vi "Sample_application.vi"() -> ()   [LabVIEW 2026]
uses:
  x64/Release/CanSharkApi_Dll1.dll
panel:
  in  "datalog":bool
  out "?":string="CAN Shark API's for Classic CAN & CANFD communication"
  in  "error in":errorcluster
  out "Serial Number":u32[](array[numeric])
  out "Device Path":string[](array[string])
  out "Connected Devices":string
  out "?":string="CAN Shark API's for Classic CAN & CANFD communication"
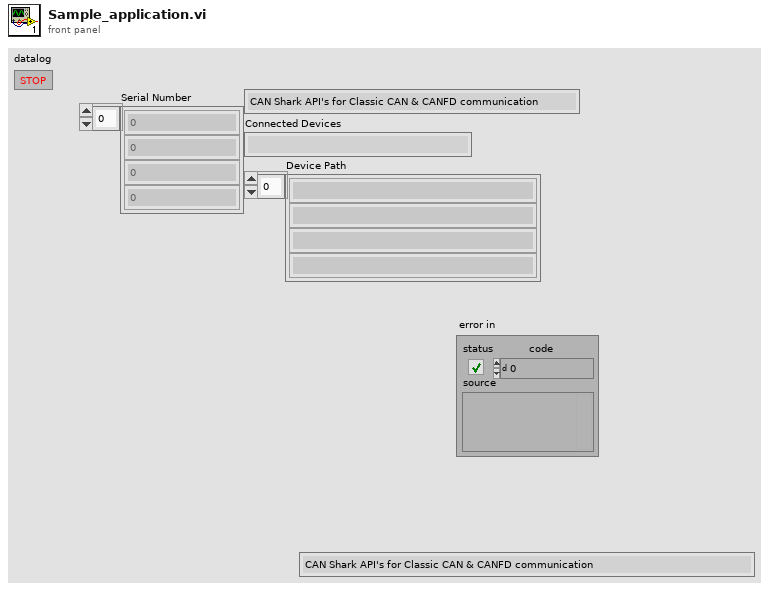
[diagram p1: front panel]
types:
  T1 = cluster{"cluster":cluster{"initialized array[0]":u16, "initialized array[1]":u16, "initialized array[2]":u16, "initialized array[3]":u16, "initialized array[4]":u16, "initialized array[5]":u16, "initialized array[6]":u16, "initialized array[7]":u16, "initialized array[8]":u16, "initialized array[9]":u16, "initialized array[10]":u16, "initialized array[11]":u16, "initialized array[12]":u16, "initialized array[13]":u16, "initialized array[14]":u16, "initialized array[15]":u16, "initialized array[16]":u16, "initialized array[17]":u16, "initialized array[18]":u16, "initialized array[19]":u16, "initialized array[20]":u16, "initialized array[21]":u16, "initialized array[22]":u16, "initialized array[23]":u16, "initialized array[24]":u16, "initialized array[25]":u16, "initialized array[26]":u16, "initialized array[27]":u16, "initialized array[28]":u16, "initialized array[29]":u16, "initialized array[30]":u16, "initialized array[31]":u16, "initialized array[32]":u16, "initialized array[33]":u16, "initialized array[34]":u16, "initialized array[35]":u16, "initialized array[36]":u16, "initialized array[37]":u16, "initialized array[38]":u16, "initialized array[39]":u16, "initialized array[40]":u16, "initialized array[41]":u16, "initialized array[42]":u16, "initialized array[43]":u16, "initialized array[44]":u16, "initialized array[45]":u16, "initialized array[46]":u16, "initialized array[47]":u16, "initialized array[48]":u16, "initialized array[49]":u16, "initialized array[50]":u16, "initialized array[51]":u16, "initialized array[52]":u16, "initialized array[53]":u16, "initialized array[54]":u16, "initialized array[55]":u16, "initialized array[56]":u16, "initialized array[57]":u16, "initialized array[58]":u16, "initialized array[59]":u16, "initialized array[60]":u16, "initialized array[61]":u16, "initialized array[62]":u16, "initialized array[63]":u16, "initialized array[64]":u16, "initialized array[65]":u16, "initialized array[66]":u16, "initialized array[67]":u16, "initialized array[68]":u16, "initialized array[69]":u16, "initialized array[70]":u16, "initialized array[71]":u16, "initialized array[72]":u16, "initialized array[73]":u16, "initialized array[74]":u16, "initialized array[75]":u16, "initialized array[76]":u16, "initialized array[77]":u16, "initialized array[78]":u16, "initialized array[79]":u16, "initialized array[80]":u16, "initialized array[81]":u16, "initialized array[82]":u16, "initialized array[83]":u16, "initialized array[84]":u16, "initialized array[85]":u16, "initialized array[86]":u16, "initialized array[87]":u16, "initialized array[88]":u16, "initialized array[89]":u16, "initialized array[90]":u16, "initialized array[91]":u16, "initialized array[92]":u16, "initialized array[93]":u16, "initialized array[94]":u16, "initialized array[95]":u16, "initialized array[96]":u16, "initialized array[97]":u16, "initialized array[98]":u16, "initialized array[99]":u16, "initialized array[100]":u16, "initialized array[101]":u16, "initialized array[102]":u16, "initialized array[103]":u16, "initialized array[104]":u16, "initialized array[105]":u16, "initialized array[106]":u16, "initialized array[107]":u16, "initialized array[108]":u16, "initialized array[109]":u16, "initialized array[110]":u16, "initialized array[111]":u16, "initialized array[112]":u16, "initialized array[113]":u16, "initialized array[114]":u16, "initialized array[115]":u16, "initialized array[116]":u16, "initialized array[117]":u16, "initialized array[118]":u16, "initialized array[119]":u16, "initialized array[120]":u16, "initialized array[121]":u16, "initialized array[122]":u16, "initialized array[123]":u16, "initialized array[124]":u16, "initialized array[125]":u16, "initialized array[126]":u16, "initialized array[127]":u16, "initialized array[128]":u16, "initialized array[129]":u16, "initialized array[130]":u16, "initialized array[131]":u16, "initialized array[132]":u16, "initialized array[133]":u16, "initialized array[134]":u16, "initialized array[135]":u16, "initialized array[136]":u16, "initialized array[137]":u16, "initialized array[138]":u16, "initialized array[139]":u16, "initialized array[140]":u16, "initialized array[141]":u16, "initialized array[142]":u16, "initialized array[143]":u16, "initialized array[144]":u16, "initialized array[145]":u16, "initialized array[146]":u16, "initialized array[147]":u16, "initialized array[148]":u16, "initialized array[149]":u16, "initialized array[150]":u16, "initialized array[151]":u16, "initialized array[152]":u16, "initialized array[153]":u16, "initialized array[154]":u16, "initialized array[155]":u16, "initialized array[156]":u16, "initialized array[157]":u16, "initialized array[158]":u16, "initialized array[159]":u16, "initialized array[160]":u16, "initialized array[161]":u16, "initialized array[162]":u16, "initialized array[163]":u16, "initialized array[164]":u16, "initialized array[165]":u16, "initialized array[166]":u16, "initialized array[167]":u16, "initialized array[168]":u16, "initialized array[169]":u16, "initialized array[170]":u16, "initialized array[171]":u16, "initialized array[172]":u16, "initialized array[173]":u16, "initialized array[174]":u16, "initialized array[175]":u16, "initialized array[176]":u16, "initialized array[177]":u16, "initialized array[178]":u16, "initialized array[179]":u16, "initialized array[180]":u16, "initialized array[181]":u16, "initialized array[182]":u16, "initialized array[183]":u16, "initialized array[184]":u16, "initialized array[185]":u16, "initialized array[186]":u16, "initialized array[187]":u16, "initialized array[188]":u16, "initialized array[189]":u16, "initialized array[190]":u16, "initialized array[191]":u16, "initialized array[192]":u16, "initialized array[193]":u16, "initialized array[194]":u16, "initialized array[195]":u16, "initialized array[196]":u16, "initialized array[197]":u16, "initialized array[198]":u16, "initialized array[199]":u16, "initialized array[200]":u16, "initialized array[201]":u16, "initialized array[202]":u16, "initialized array[203]":u16, "initialized array[204]":u16, "initialized array[205]":u16, "initialized array[206]":u16, "initialized array[207]":u16, "initialized array[208]":u16, "initialized array[209]":u16, "initialized array[210]":u16, "initialized array[211]":u16, "initialized array[212]":u16, "initialized array[213]":u16, "initialized array[214]":u16, "initialized array[215]":u16, "initialized array[216]":u16, "initialized array[217]":u16, "initialized array[218]":u16, "initialized array[219]":u16, "initialized array[220]":u16, "initialized array[221]":u16, "initialized array[222]":u16, "initialized array[223]":u16, "initialized array[224]":u16, "initialized array[225]":u16, "initialized array[226]":u16, "initialized array[227]":u16, "initialized array[228]":u16, "initialized array[229]":u16, "initialized array[230]":u16, "initialized array[231]":u16, "initialized array[232]":u16, "initialized array[233]":u16, "initialized array[234]":u16, "initialized array[235]":u16, "initialized array[236]":u16, "initialized array[237]":u16, "initialized array[238]":u16, "initialized array[239]":u16, "initialized array[240]":u16, "initialized array[241]":u16, "initialized array[242]":u16, "initialized array[243]":u16, "initialized array[244]":u16, "initialized array[245]":u16, "initialized array[246]":u16, "initialized array[247]":u16, "initialized array[248]":u16, "initialized array[249]":u16, "initialized array[250]":u16, "initialized array[251]":u16, "initialized array[252]":u16, "initialized array[253]":u16, "initialized array[254]":u16, "initialized array[255]":u16}, "Serial Number":u32}[]
  T2 = cluster{"cluster":cluster{"initialized array[0]":u16, "initialized array[1]":u16, "initialized array[2]":u16, "initialized array[3]":u16, "initialized array[4]":u16, "initialized array[5]":u16, "initialized array[6]":u16, "initialized array[7]":u16, "initialized array[8]":u16, "initialized array[9]":u16, "initialized array[10]":u16, "initialized array[11]":u16, "initialized array[12]":u16, "initialized array[13]":u16, "initialized array[14]":u16, "initialized array[15]":u16, "initialized array[16]":u16, "initialized array[17]":u16, "initialized array[18]":u16, "initialized array[19]":u16, "initialized array[20]":u16, "initialized array[21]":u16, "initialized array[22]":u16, "initialized array[23]":u16, "initialized array[24]":u16, "initialized array[25]":u16, "initialized array[26]":u16, "initialized array[27]":u16, "initialized array[28]":u16, "initialized array[29]":u16, "initialized array[30]":u16, "initialized array[31]":u16, "initialized array[32]":u16, "initialized array[33]":u16, "initialized array[34]":u16, "initialized array[35]":u16, "initialized array[36]":u16, "initialized array[37]":u16, "initialized array[38]":u16, "initialized array[39]":u16, "initialized array[40]":u16, "initialized array[41]":u16, "initialized array[42]":u16, "initialized array[43]":u16, "initialized array[44]":u16, "initialized array[45]":u16, "initialized array[46]":u16, "initialized array[47]":u16, "initialized array[48]":u16, "initialized array[49]":u16, "initialized array[50]":u16, "initialized array[51]":u16, "initialized array[52]":u16, "initialized array[53]":u16, "initialized array[54]":u16, "initialized array[55]":u16, "initialized array[56]":u16, "initialized array[57]":u16, "initialized array[58]":u16, "initialized array[59]":u16, "initialized array[60]":u16, "initialized array[61]":u16, "initialized array[62]":u16, "initialized array[63]":u16, "initialized array[64]":u16, "initialized array[65]":u16, "initialized array[66]":u16, "initialized array[67]":u16, "initialized array[68]":u16, "initialized array[69]":u16, "initialized array[70]":u16, "initialized array[71]":u16, "initialized array[72]":u16, "initialized array[73]":u16, "initialized array[74]":u16, "initialized array[75]":u16, "initialized array[76]":u16, "initialized array[77]":u16, "initialized array[78]":u16, "initialized array[79]":u16, "initialized array[80]":u16, "initialized array[81]":u16, "initialized array[82]":u16, "initialized array[83]":u16, "initialized array[84]":u16, "initialized array[85]":u16, "initialized array[86]":u16, "initialized array[87]":u16, "initialized array[88]":u16, "initialized array[89]":u16, "initialized array[90]":u16, "initialized array[91]":u16, "initialized array[92]":u16, "initialized array[93]":u16, "initialized array[94]":u16, "initialized array[95]":u16, "initialized array[96]":u16, "initialized array[97]":u16, "initialized array[98]":u16, "initialized array[99]":u16, "initialized array[100]":u16, "initialized array[101]":u16, "initialized array[102]":u16, "initialized array[103]":u16, "initialized array[104]":u16, "initialized array[105]":u16, "initialized array[106]":u16, "initialized array[107]":u16, "initialized array[108]":u16, "initialized array[109]":u16, "initialized array[110]":u16, "initialized array[111]":u16, "initialized array[112]":u16, "initialized array[113]":u16, "initialized array[114]":u16, "initialized array[115]":u16, "initialized array[116]":u16, "initialized array[117]":u16, "initialized array[118]":u16, "initialized array[119]":u16, "initialized array[120]":u16, "initialized array[121]":u16, "initialized array[122]":u16, "initialized array[123]":u16, "initialized array[124]":u16, "initialized array[125]":u16, "initialized array[126]":u16, "initialized array[127]":u16, "initialized array[128]":u16, "initialized array[129]":u16, "initialized array[130]":u16, "initialized array[131]":u16, "initialized array[132]":u16, "initialized array[133]":u16, "initialized array[134]":u16, "initialized array[135]":u16, "initialized array[136]":u16, "initialized array[137]":u16, "initialized array[138]":u16, "initialized array[139]":u16, "initialized array[140]":u16, "initialized array[141]":u16, "initialized array[142]":u16, "initialized array[143]":u16, "initialized array[144]":u16, "initialized array[145]":u16, "initialized array[146]":u16, "initialized array[147]":u16, "initialized array[148]":u16, "initialized array[149]":u16, "initialized array[150]":u16, "initialized array[151]":u16, "initialized array[152]":u16, "initialized array[153]":u16, "initialized array[154]":u16, "initialized array[155]":u16, "initialized array[156]":u16, "initialized array[157]":u16, "initialized array[158]":u16, "initialized array[159]":u16, "initialized array[160]":u16, "initialized array[161]":u16, "initialized array[162]":u16, "initialized array[163]":u16, "initialized array[164]":u16, "initialized array[165]":u16, "initialized array[166]":u16, "initialized array[167]":u16, "initialized array[168]":u16, "initialized array[169]":u16, "initialized array[170]":u16, "initialized array[171]":u16, "initialized array[172]":u16, "initialized array[173]":u16, "initialized array[174]":u16, "initialized array[175]":u16, "initialized array[176]":u16, "initialized array[177]":u16, "initialized array[178]":u16, "initialized array[179]":u16, "initialized array[180]":u16, "initialized array[181]":u16, "initialized array[182]":u16, "initialized array[183]":u16, "initialized array[184]":u16, "initialized array[185]":u16, "initialized array[186]":u16, "initialized array[187]":u16, "initialized array[188]":u16, "initialized array[189]":u16, "initialized array[190]":u16, "initialized array[191]":u16, "initialized array[192]":u16, "initialized array[193]":u16, "initialized array[194]":u16, "initialized array[195]":u16, "initialized array[196]":u16, "initialized array[197]":u16, "initialized array[198]":u16, "initialized array[199]":u16, "initialized array[200]":u16, "initialized array[201]":u16, "initialized array[202]":u16, "initialized array[203]":u16, "initialized array[204]":u16, "initialized array[205]":u16, "initialized array[206]":u16, "initialized array[207]":u16, "initialized array[208]":u16, "initialized array[209]":u16, "initialized array[210]":u16, "initialized array[211]":u16, "initialized array[212]":u16, "initialized array[213]":u16, "initialized array[214]":u16, "initialized array[215]":u16, "initialized array[216]":u16, "initialized array[217]":u16, "initialized array[218]":u16, "initialized array[219]":u16, "initialized array[220]":u16, "initialized array[221]":u16, "initialized array[222]":u16, "initialized array[223]":u16, "initialized array[224]":u16, "initialized array[225]":u16, "initialized array[226]":u16, "initialized array[227]":u16, "initialized array[228]":u16, "initialized array[229]":u16, "initialized array[230]":u16, "initialized array[231]":u16, "initialized array[232]":u16, "initialized array[233]":u16, "initialized array[234]":u16, "initialized array[235]":u16, "initialized array[236]":u16, "initialized array[237]":u16, "initialized array[238]":u16, "initialized array[239]":u16, "initialized array[240]":u16, "initialized array[241]":u16, "initialized array[242]":u16, "initialized array[243]":u16, "initialized array[244]":u16, "initialized array[245]":u16, "initialized array[246]":u16, "initialized array[247]":u16, "initialized array[248]":u16, "initialized array[249]":u16, "initialized array[250]":u16, "initialized array[251]":u16, "initialized array[252]":u16, "initialized array[253]":u16, "initialized array[254]":u16, "initialized array[255]":u16}, "Serial Number":u32}
  T3 = cluster{"initialized array[0]":u16, "initialized array[1]":u16, "initialized array[2]":u16, "initialized array[3]":u16, "initialized array[4]":u16, "initialized array[5]":u16, "initialized array[6]":u16, "initialized array[7]":u16, "initialized array[8]":u16, "initialized array[9]":u16, "initialized array[10]":u16, "initialized array[11]":u16, "initialized array[12]":u16, "initialized array[13]":u16, "initialized array[14]":u16, "initialized array[15]":u16, "initialized array[16]":u16, "initialized array[17]":u16, "initialized array[18]":u16, "initialized array[19]":u16, "initialized array[20]":u16, "initialized array[21]":u16, "initialized array[22]":u16, "initialized array[23]":u16, "initialized array[24]":u16, "initialized array[25]":u16, "initialized array[26]":u16, "initialized array[27]":u16, "initialized array[28]":u16, "initialized array[29]":u16, "initialized array[30]":u16, "initialized array[31]":u16, "initialized array[32]":u16, "initialized array[33]":u16, "initialized array[34]":u16, "initialized array[35]":u16, "initialized array[36]":u16, "initialized array[37]":u16, "initialized array[38]":u16, "initialized array[39]":u16, "initialized array[40]":u16, "initialized array[41]":u16, "initialized array[42]":u16, "initialized array[43]":u16, "initialized array[44]":u16, "initialized array[45]":u16, "initialized array[46]":u16, "initialized array[47]":u16, "initialized array[48]":u16, "initialized array[49]":u16, "initialized array[50]":u16, "initialized array[51]":u16, "initialized array[52]":u16, "initialized array[53]":u16, "initialized array[54]":u16, "initialized array[55]":u16, "initialized array[56]":u16, "initialized array[57]":u16, "initialized array[58]":u16, "initialized array[59]":u16, "initialized array[60]":u16, "initialized array[61]":u16, "initialized array[62]":u16, "initialized array[63]":u16, "initialized array[64]":u16, "initialized array[65]":u16, "initialized array[66]":u16, "initialized array[67]":u16, "initialized array[68]":u16, "initialized array[69]":u16, "initialized array[70]":u16, "initialized array[71]":u16, "initialized array[72]":u16, "initialized array[73]":u16, "initialized array[74]":u16, "initialized array[75]":u16, "initialized array[76]":u16, "initialized array[77]":u16, "initialized array[78]":u16, "initialized array[79]":u16, "initialized array[80]":u16, "initialized array[81]":u16, "initialized array[82]":u16, "initialized array[83]":u16, "initialized array[84]":u16, "initialized array[85]":u16, "initialized array[86]":u16, "initialized array[87]":u16, "initialized array[88]":u16, "initialized array[89]":u16, "initialized array[90]":u16, "initialized array[91]":u16, "initialized array[92]":u16, "initialized array[93]":u16, "initialized array[94]":u16, "initialized array[95]":u16, "initialized array[96]":u16, "initialized array[97]":u16, "initialized array[98]":u16, "initialized array[99]":u16, "initialized array[100]":u16, "initialized array[101]":u16, "initialized array[102]":u16, "initialized array[103]":u16, "initialized array[104]":u16, "initialized array[105]":u16, "initialized array[106]":u16, "initialized array[107]":u16, "initialized array[108]":u16, "initialized array[109]":u16, "initialized array[110]":u16, "initialized array[111]":u16, "initialized array[112]":u16, "initialized array[113]":u16, "initialized array[114]":u16, "initialized array[115]":u16, "initialized array[116]":u16, "initialized array[117]":u16, "initialized array[118]":u16, "initialized array[119]":u16, "initialized array[120]":u16, "initialized array[121]":u16, "initialized array[122]":u16, "initialized array[123]":u16, "initialized array[124]":u16, "initialized array[125]":u16, "initialized array[126]":u16, "initialized array[127]":u16, "initialized array[128]":u16, "initialized array[129]":u16, "initialized array[130]":u16, "initialized array[131]":u16, "initialized array[132]":u16, "initialized array[133]":u16, "initialized array[134]":u16, "initialized array[135]":u16, "initialized array[136]":u16, "initialized array[137]":u16, "initialized array[138]":u16, "initialized array[139]":u16, "initialized array[140]":u16, "initialized array[141]":u16, "initialized array[142]":u16, "initialized array[143]":u16, "initialized array[144]":u16, "initialized array[145]":u16, "initialized array[146]":u16, "initialized array[147]":u16, "initialized array[148]":u16, "initialized array[149]":u16, "initialized array[150]":u16, "initialized array[151]":u16, "initialized array[152]":u16, "initialized array[153]":u16, "initialized array[154]":u16, "initialized array[155]":u16, "initialized array[156]":u16, "initialized array[157]":u16, "initialized array[158]":u16, "initialized array[159]":u16, "initialized array[160]":u16, "initialized array[161]":u16, "initialized array[162]":u16, "initialized array[163]":u16, "initialized array[164]":u16, "initialized array[165]":u16, "initialized array[166]":u16, "initialized array[167]":u16, "initialized array[168]":u16, "initialized array[169]":u16, "initialized array[170]":u16, "initialized array[171]":u16, "initialized array[172]":u16, "initialized array[173]":u16, "initialized array[174]":u16, "initialized array[175]":u16, "initialized array[176]":u16, "initialized array[177]":u16, "initialized array[178]":u16, "initialized array[179]":u16, "initialized array[180]":u16, "initialized array[181]":u16, "initialized array[182]":u16, "initialized array[183]":u16, "initialized array[184]":u16, "initialized array[185]":u16, "initialized array[186]":u16, "initialized array[187]":u16, "initialized array[188]":u16, "initialized array[189]":u16, "initialized array[190]":u16, "initialized array[191]":u16, "initialized array[192]":u16, "initialized array[193]":u16, "initialized array[194]":u16, "initialized array[195]":u16, "initialized array[196]":u16, "initialized array[197]":u16, "initialized array[198]":u16, "initialized array[199]":u16, "initialized array[200]":u16, "initialized array[201]":u16, "initialized array[202]":u16, "initialized array[203]":u16, "initialized array[204]":u16, "initialized array[205]":u16, "initialized array[206]":u16, "initialized array[207]":u16, "initialized array[208]":u16, "initialized array[209]":u16, "initialized array[210]":u16, "initialized array[211]":u16, "initialized array[212]":u16, "initialized array[213]":u16, "initialized array[214]":u16, "initialized array[215]":u16, "initialized array[216]":u16, "initialized array[217]":u16, "initialized array[218]":u16, "initialized array[219]":u16, "initialized array[220]":u16, "initialized array[221]":u16, "initialized array[222]":u16, "initialized array[223]":u16, "initialized array[224]":u16, "initialized array[225]":u16, "initialized array[226]":u16, "initialized array[227]":u16, "initialized array[228]":u16, "initialized array[229]":u16, "initialized array[230]":u16, "initialized array[231]":u16, "initialized array[232]":u16, "initialized array[233]":u16, "initialized array[234]":u16, "initialized array[235]":u16, "initialized array[236]":u16, "initialized array[237]":u16, "initialized array[238]":u16, "initialized array[239]":u16, "initialized array[240]":u16, "initialized array[241]":u16, "initialized array[242]":u16, "initialized array[243]":u16, "initialized array[244]":u16, "initialized array[245]":u16, "initialized array[246]":u16, "initialized array[247]":u16, "initialized array[248]":u16, "initialized array[249]":u16, "initialized array[250]":u16, "initialized array[251]":u16, "initialized array[252]":u16, "initialized array[253]":u16, "initialized array[254]":u16, "initialized array[255]":u16}
  T4 = cluster{"DeviceIndex":i32, "Mode":i32, "BaudRate":i32, "DataBitRate":i32}[]
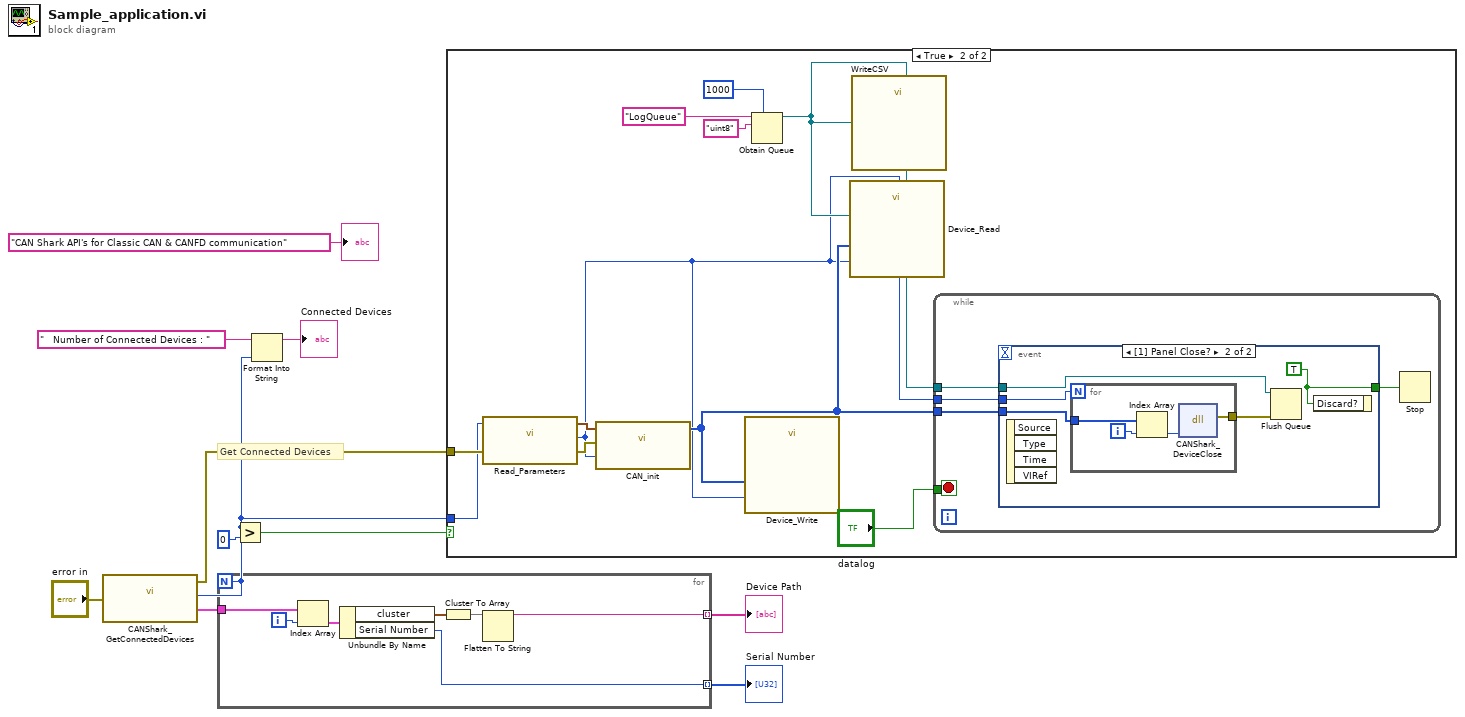
[diagram p0: block diagram]
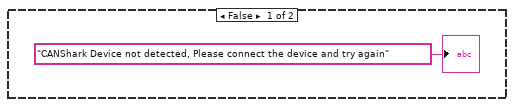
[diagram p2: hidden frame]
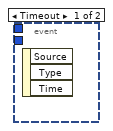
[diagram p3: hidden frame]
diagram:
  # "Get Connected Devices"
  n1 = call "CANShark_GetConnectedDevices.vi"("error in (no error)"="error in") -> ("deviceList"=w5:T1, "Connected Devices"=w1:u8, "error out"=w3:errorcluster)  [unwired: 8 in]
  n2 = for {
    N: w1 -> [_]
    tunnel: [w15] -> w7 mode=indexing
    tunnel: [w14] -> w8 mode=indexing
    tunnel: w5 -> [w12]
    i -> [w18]
    n3 = Index Array(array=w12, index=w18) -> (element=w13:T2)
    n4 = Unbundle By Name(w13) -> ("cluster"=w17:T3, "Serial Number"=w15:u32)
    n5 = Cluster To Array(cluster=w17) -> (array=w16:u16[])
    n6 = Flatten To String(anything=w16) -> (data string=w14:string)  [unwired: 3 in, 2 out]
  }
  "Device Path" <- w8
  "Serial Number" <- w7
  n7 = Greater?(x=w1, y=u8 0) -> (0:w2:bool)
  n8 = Format Into String(initial string="   Number of Connected Devices : ", w1) -> (resulting string=→"Connected Devices":string)  [unwired: 2 in, 1 out]
  n9 = case shown="True" w2 {
    tunnel: w3 -> [_ w28]
    tunnel: w1 -> [_ w27]
    frame False {
      "?" <- "CANShark Device not detected, Please connect the device and try again"
    }
    frame True {
      n10 = call "Read_Parameters.vi"("error in"=w28, "device count"=w27) -> ("error out"=w29:errorcluster, "Selected Devices"=w20:i32, "Device Configuration"=w30:T4)  [unwired: 7 in]
      n11 = call "CAN_init.vi"("Selected Count"=w20, "error in (no error)"=w29, "DEVICE CONFIG"=w30) -> ("Device Handler"=w25:i64[])  [unwired: 7 in, 1 out]
      n12 = call "Device_Write.vi"("Device Handler pointers"=w25, "Selected Device count"=w20) -> ()  [unwired: 10 in]
      n13 = Obtain Queue(max queue size (-1, unlimited)=1000, name (unnamed)="LogQueue", element data type="uint8") -> (queue out=w21:refnum<queue>)  [unwired: 2 in, 2 out]
      n14 = call "Device_Read.vi"("queue out"=w21, "Selected Count"=w20, "Device Handler pointer"=w25) -> ()  [unwired: 9 in]
      n15 = call "WriteCSV.vi"("Log Queue"=w21) -> ()  [unwired: 9 in, 2 out]
      n16 = while {
        tunnel: w25 -> [w35]
        tunnel: w20 -> [w34]
        tunnel: "datalog" -> [w33]
        tunnel: w21 -> [w31]
        stop <- w33 stop-if-true
        n17 = event shown="[1] Panel Close?" {
          selector: _ -> [_ _]
          dyn-events: _ -> [_ _]
          timeout: _ -> [_ _]
          tunnel: w35 -> [_ w39]
          tunnel: w34 -> [_ w40]
          tunnel: [_ w38] -> w32
          tunnel: w31 -> [_ w36]
          event Timeout {
            n18 = event-data() -> ()  [unwired: 1 in, 3 out]
          }
          event Panel Close? {
            w38 = TRUE
            n19 = event-data() -> ()  [unwired: 1 in, 4 out]
            n20 = for {
              N: w40 -> [_]
              tunnel: w39 -> [w42]
              tunnel: [w41] -> w37
              i -> [w43]
              n21 = Index Array(array=w42, index=w43) -> (element=w44:i64)
              n22 = dll-call lib="C:/Users/TECQNIO/Documents/CANSHARK LABVIEW API PACKAGE/x64/Release/CanSharkApi_Dll1.dll" fn="CANShark_DeviceClose"("Device"=w44) -> (error out=w41:errorcluster)  [unwired: 5 in, 1 out]
            }
            n23 = Flush Queue(queue=w36, error in (no error)=w37) -> ()  [unwired: 3 out]
            n24 = event-data("Discard?"=w38) -> ()  [unwired: 1 in, 1 out]
          }
        }
        n25 = Stop(stop? (T)=w32) -> ()
      }
    }
  }
  "?" <- "CAN Shark API's for Classic CAN & CANFD communication"
